vi "SM_CaseSelect.vi"(11 "Input":string[](array[string])) -> (3 "Case":string)   [LabVIEW 2022 SP3]
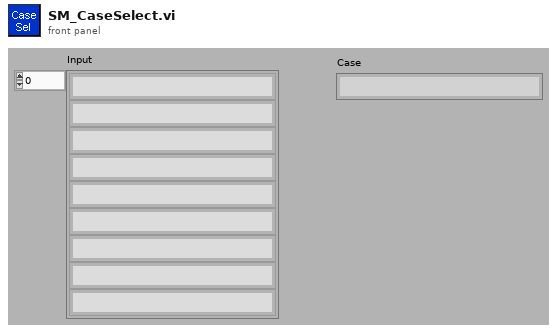
[diagram p1: front panel]
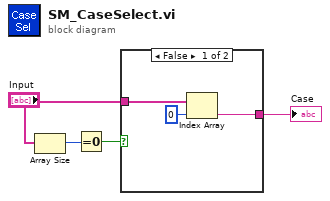
[diagram p0: block diagram]
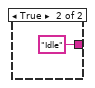
[diagram p2: hidden frame]
diagram:
  n1 = Array Size(array="Input") -> (size(s)=w2:i32)
  n2 = Equal To 0?(x=w2) -> (x = 0?=w1:bool)
  n3 = case shown="False" w1 {
    tunnel: [w6 "Idle" ("文字列")] -> w4
    tunnel: "Input" -> [w5 _]
    frame False {
      n4 = Index Array(array=w5, index=0 ("指標")) -> (element=w6:string)
    }
    frame True {
    }
  }
  "Case" <- w4
